vi "Convert Channels to Configuration.vi"(8 "error in":errorcluster, 10 "Conversion time":u16, 11 "Channels":T2(array[cluster])) -> (0 "error out":errorcluster, 3 "_9216 Config Data":T1)   [LabVIEW 2017, in "Modules.lvlib" / "9216.lvclass"]
uses:
  9216.lvclass
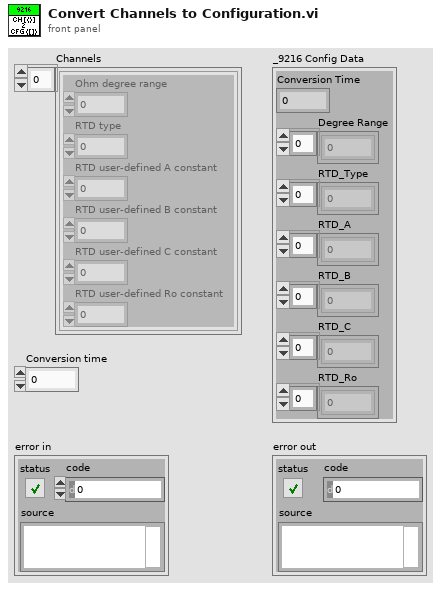
[diagram p1: front panel]
types:
  T1 = cluster{"Conversion Time":u16, "Degree Range":u8[], "RTD_Type":u8[], "RTD_A":dbl[], "RTD_B":dbl[], "RTD_C":dbl[], "RTD_Ro":dbl[]}
  T2 = cluster{"Ohm degree range":u32, "RTD type":u32, "RTD user-defined A constant":dbl, "RTD user-defined B constant":dbl, "RTD user-defined C constant":dbl, "RTD user-defined Ro constant":dbl}[]
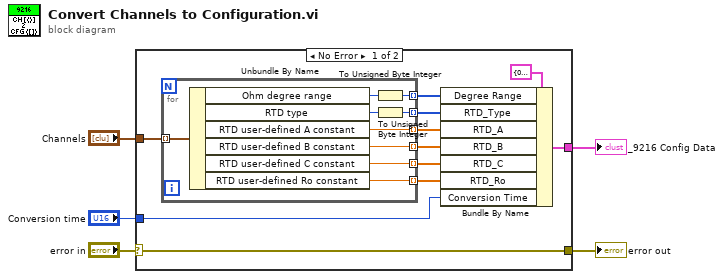
[diagram p0: block diagram]
diagram:
  n1 = case shown="No Error" "error in" {
    selector: "error in" -> [w7 w26]
    tunnel: [w7 w26] -> w3
    tunnel: "Channels" -> [w15 _]
    tunnel: "Conversion time" -> [w6 _]
    tunnel: [w8 _] -> w4
    frame No Error {
      n2 = for {
        tunnel: w15 -> [w25] mode=indexing
        tunnel: [w18] -> w14 mode=indexing
        tunnel: [w17] -> w13 mode=indexing
        tunnel: [w22] -> w12 mode=indexing
        tunnel: [w21] -> w11 mode=indexing
        tunnel: [w20] -> w10 mode=indexing
        tunnel: [w19] -> w9 mode=indexing
        n3 = Unbundle By Name(w25) -> ("Ohm degree range"=w24:u32, "RTD type"=w23:u32, "RTD user-defined A constant"=w22:dbl, "RTD user-defined B constant"=w21:dbl, "RTD user-defined C constant"=w20:dbl, "RTD user-defined Ro constant"=w19:dbl)
        n4 = To Unsigned Byte Integer(number=w24) -> (unsigned 8bit integer=w18:u8)
        n5 = To Unsigned Byte Integer(number=w23) -> (unsigned 8bit integer=w17:u8)
      }
      n6 = Bundle By Name(cluster=T1 {"Conversion Time"=0, "Degree Range"=[], "RTD_Type"=[1], "RTD_A"=[], "RTD_B"=[], "RTD_C"=[], "RTD_Ro"=[]} ("_9217 Config Data"), "Degree Range"=w14, "RTD_Type"=w13, "RTD_A"=w12, "RTD_B"=w11, "RTD_C"=w10, "RTD_Ro"=w9, "Conversion Time"=w6) -> (w8:T1)
    }
    frame Error {
    }
  }
  "_9216 Config Data" <- w4
  "error out" <- w3
